vi "BratWaitForPanelClose.vi"   [LabVIEW 2012]
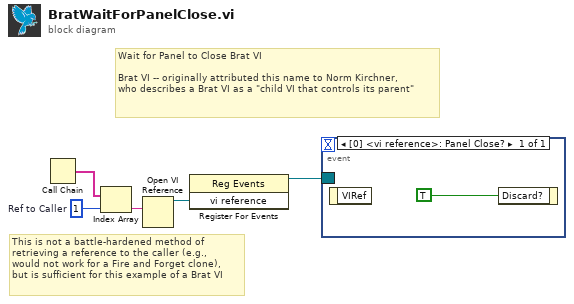
[diagram p0: block diagram]
diagram:
  w4 = 1  # Ref to Caller
  # "Wait for Panel to Close Brat VI\n\nBrat VI -- originally attributed this name to Norm Kirchner,\nwho describes a Brat VI as a \"child VI that controls its parent\""
  # "This is not a battle-hardened method of\nretrieving a reference to the caller (e.g.,\nwould not work for a Fire and Forget clone),\nbut is sufficient for this example of a Brat VI"
  n1 = Call Chain() -> (call chain=w5:string[])
  n2 = Index Array(array=w5, index=w4) -> (element=w3:string)
  n3 = Open VI Reference(vi path=w3) -> (vi reference=w2:refnum<vi>)  [unwired: 5 in, 1 out]
  n4 = register-events(w2) -> (reference out=w1:refnum<event-registration>)  [unwired: 2 in, 1 out]
  n5 = event shown="[0] <vi reference>: Panel Close?" {
    selector: w1 -> [_]
    dyn-events: _ -> [_]
    timeout: _ -> [_]
    event Panel Close? {
      n6 = event-data() -> ()  [unwired: 1 in, 1 out]
      n7 = event-data("Discard?"=TRUE) -> ()  [unwired: 1 in, 1 out]
    }
  }
